vi "get log file name.vi"() -> (0 "log file name (excluding extension)":string)   [LabVIEW 2020, in "app_log.lvlib"]
uses:
  app_log.lvlib
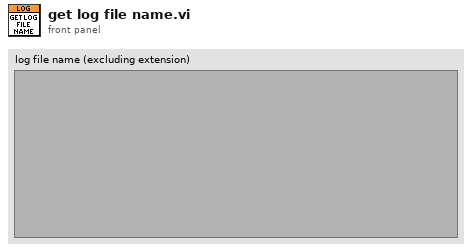
[diagram p1: front panel]
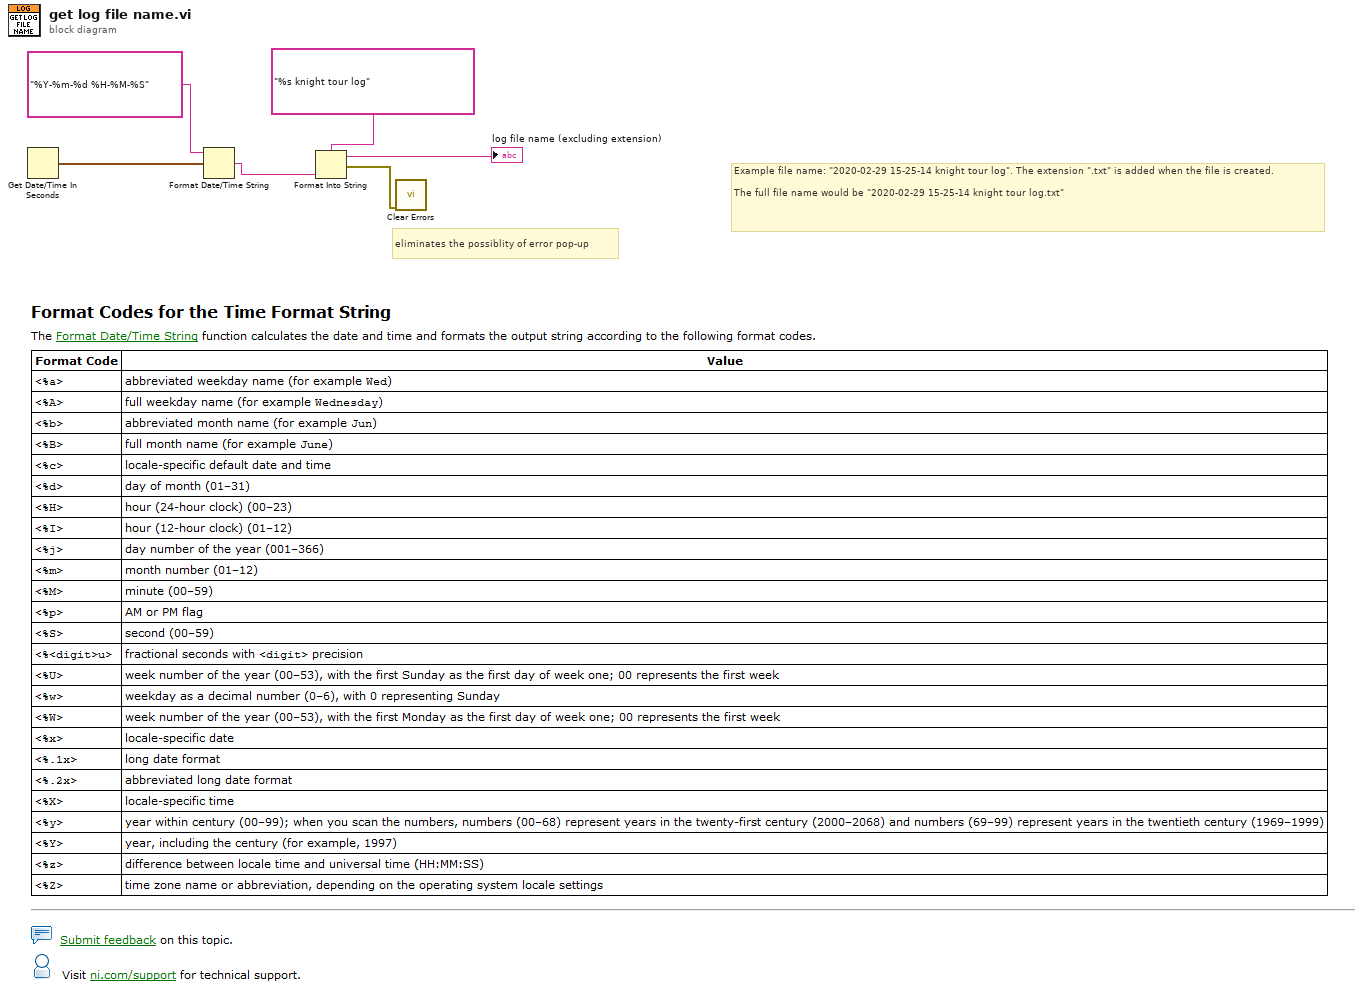
[diagram p0: block diagram]
diagram:
  # "Example file name: \"2020-02-29 15-25-14 knight tour log\". The extension \".txt\" is added when the file is created. \n\nThe full file name would be \"2020-02-29 15-25-14 knight tour log.txt\""
  # "eliminates the possiblity of error pop-up"
  n1 = Get Date/Time In Seconds() -> (seconds since 1Jan1904=w6:timestamp)
  n2 = Format Date/Time String(time format string (%c)="%Y-%m-%d %H-%M-%S", seconds (now)=w6) -> (date/time string=w2:string)  [unwired: 1 in]
  n3 = Format Into String(format string="%s knight tour log" ("time format string (%c)"), w2) -> (resulting string=→"log file name (excluding extension)":string, error out=w3:errorcluster)  [unwired: 2 in]
  n4 = call <vilib>:"Clear Errors.vi"("error in (no error)"=w3) -> ()  [unwired: 5 in, 2 out]
